vi "Main.vi"(8 "error in (no error)":errorcluster caption="错误输入（无错误）", 11 "人体监测系统 输入":refnum<class "人体健康监测系统.lvclass">) -> (0 "error out":errorcluster caption="错误输出", 3 "人体监测系统 输出":refnum<class "人体健康监测系统.lvclass">)   [LabVIEW 2020, in "人体健康监测系统.lvclass"]
uses:
  OpenUI(Setting).vi
  <vilib>/GPower/VILauncher/Library/Open/OpenByRefnumAndRunFP.vi
  <vilib>/GPower/VILauncher/VILauncher.lvlib
panel:
  in  "OK":bool
  in  "Title":bool
  in  "Title-通讯参数":string="通讯参数"
  out "通讯状态":bool
  in  "Settings":bool
  in  "Title-当前状态":string
  in  "当前状态":string
  in  "Title-模式切换":string="模式切换"
  in  "模式切换":bool
  in  "Title-参数设置":string="参数设置"
  in  "加":bool
  in  "减":bool
  in  "参数设置":bool
  in  "Title-开关机":string="开关机"
  in  "关机":bool
  in  "Title-数据采集和回放":string="数据采集和回放"
  in  "回放文件选择":path
  in  "数据回放":bool
  in  "保存文件名称":string
  in  "停止采集":bool
  in  "开始采集":bool
  out "数据曲线图":waveform(sgl)[](graph)
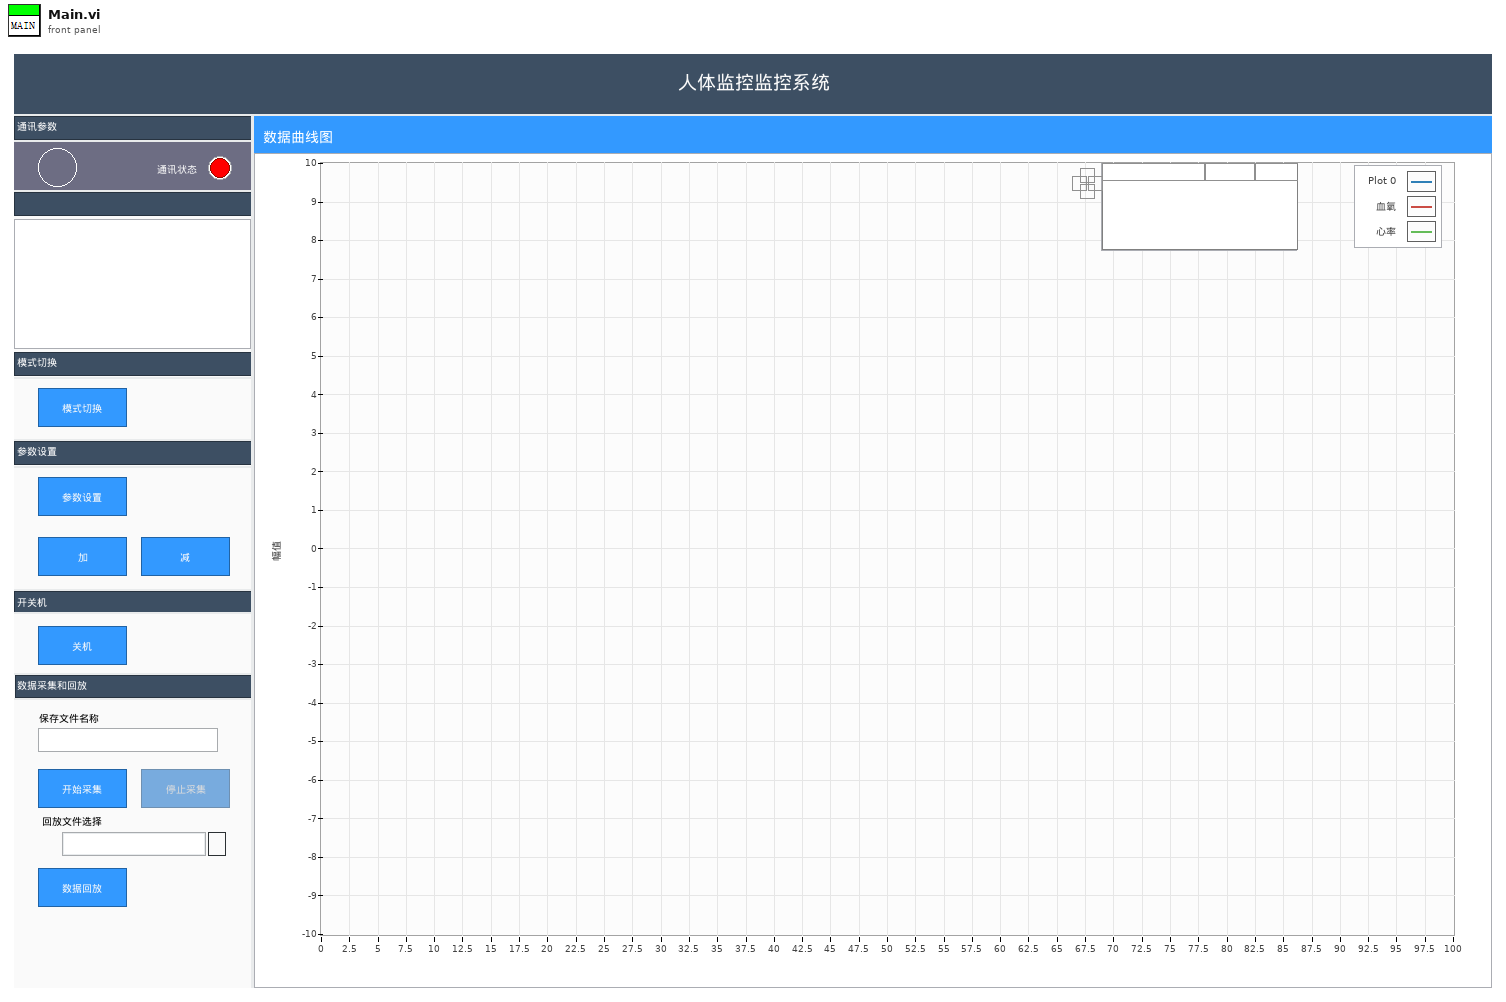
[diagram p1: front panel]
types:
  T1 = enum8{"Enabled", "Disabled", "Disabled and Grayed Out"}
  T2 = enum32{"Invalid", "Standard", "Closed", "Hidden", "Minimized", "Maximized"}
  T3 = enum32{"invalid app kind", "Development System", "Run Time System", "Student Edition", "Embedded LabVIEW", "Evaluation", "Custom"}
  T4 = cluster{"Core":cluster{"Current VI Reference":refnum<vi>, "Close Panel on Exit?":bool}, "Your Boolean data":bool, "Your string data":string, "通讯状态":refnum<vi>, "数据曲线图":refnum<vi>, "Data":waveform(sgl)[], "测试状态？":bool, "开始采集":refnum<vi>, "停止采集":refnum<vi>, "最近三次读取缓存":string[]}
  T5 = cluster{"Current VI Reference":refnum<vi>, "Close Panel on Exit?":bool}
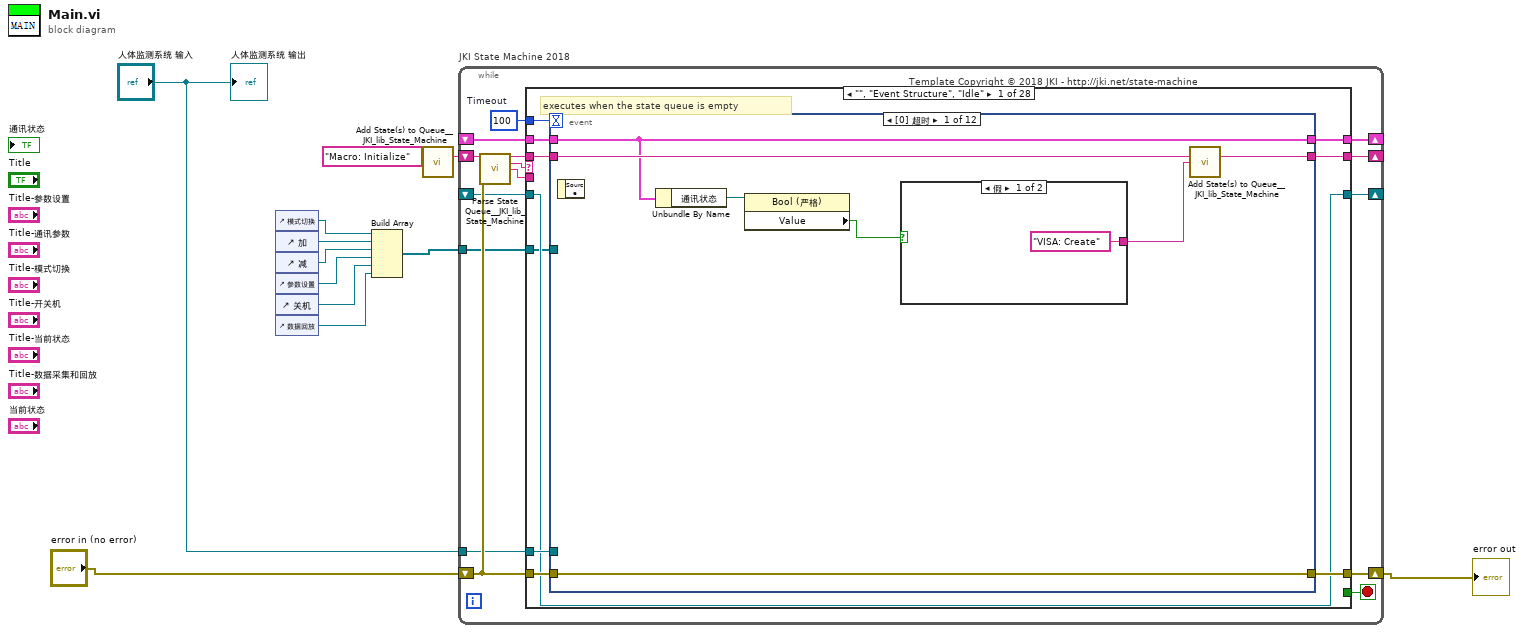
[diagram p0: block diagram]
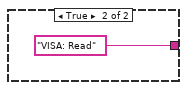
[diagram p2: hidden frame]
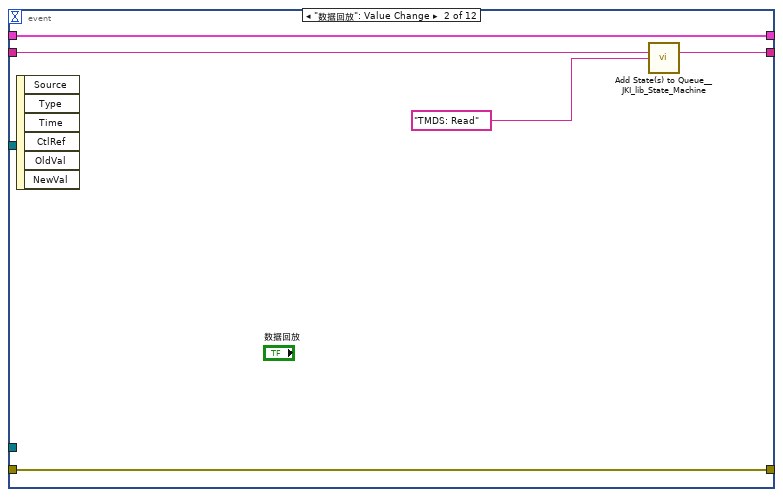
[diagram p3: hidden frame]
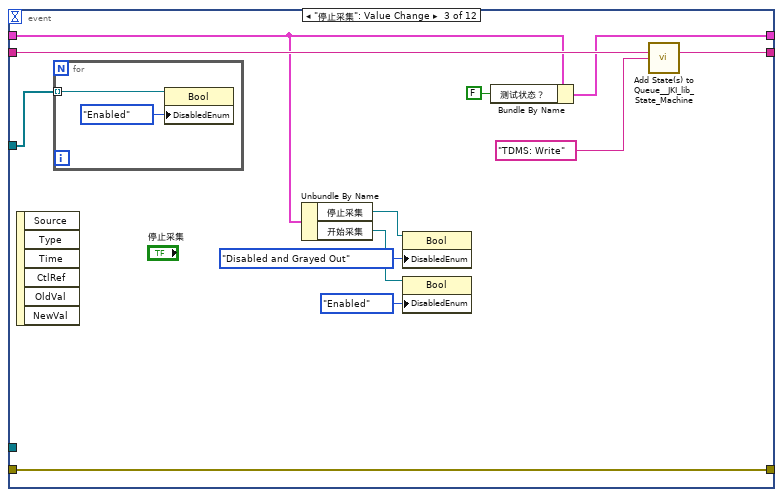
[diagram p4: hidden frame]
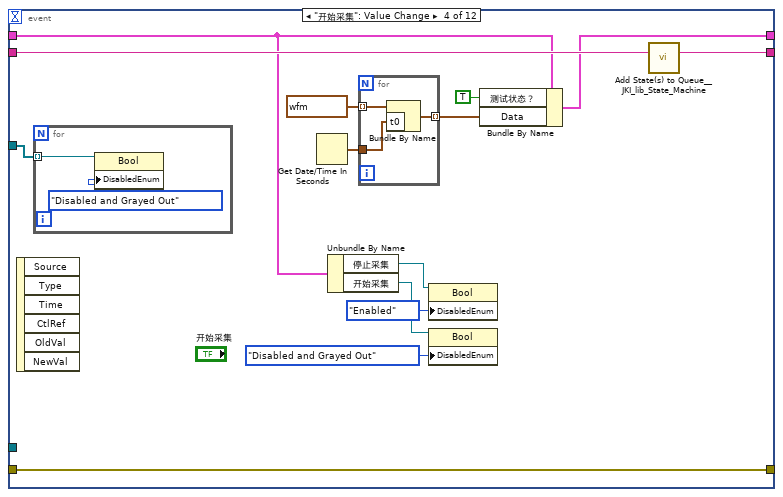
[diagram p5: hidden frame]
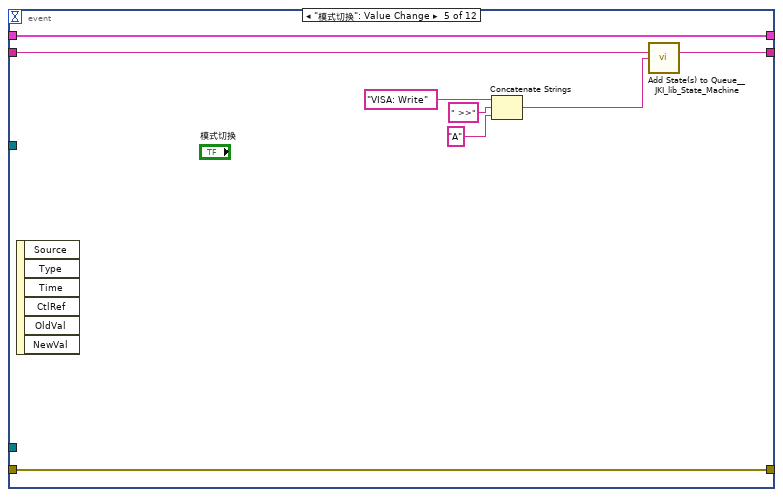
[diagram p6: hidden frame]
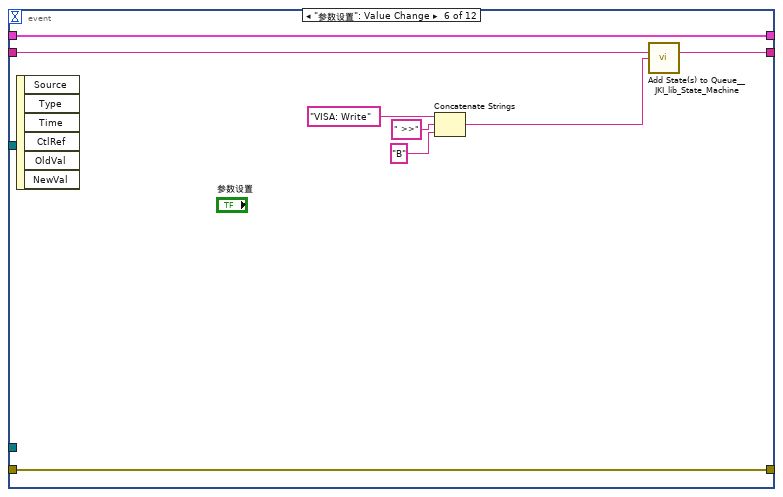
[diagram p7: hidden frame]
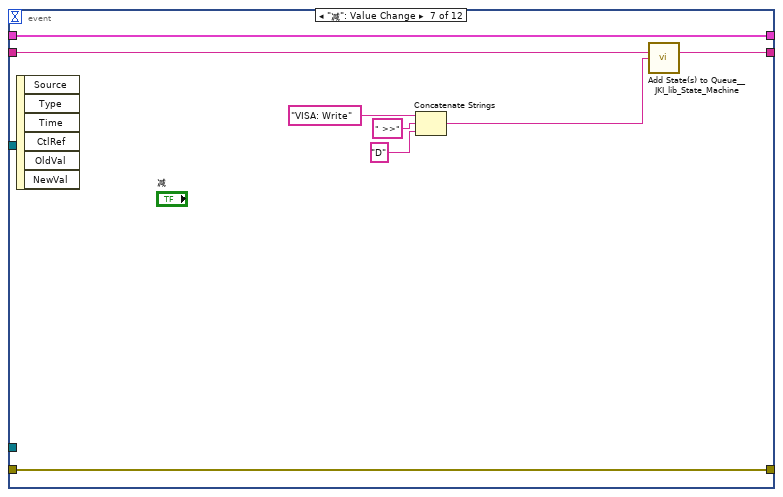
[diagram p8: hidden frame]
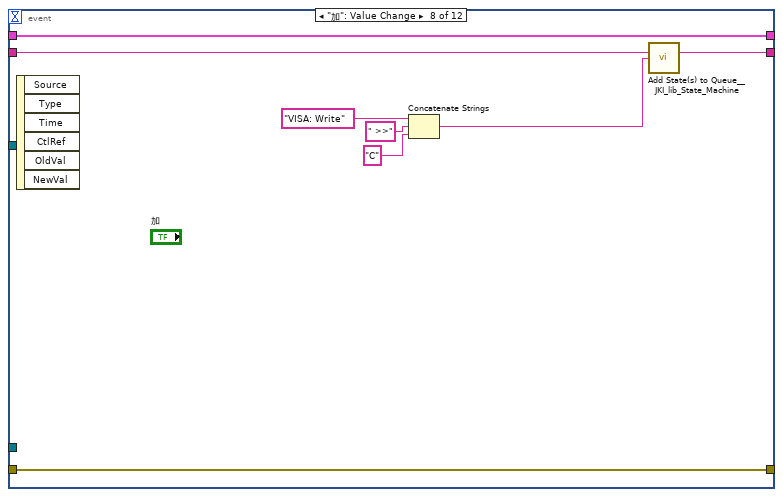
[diagram p9: hidden frame]
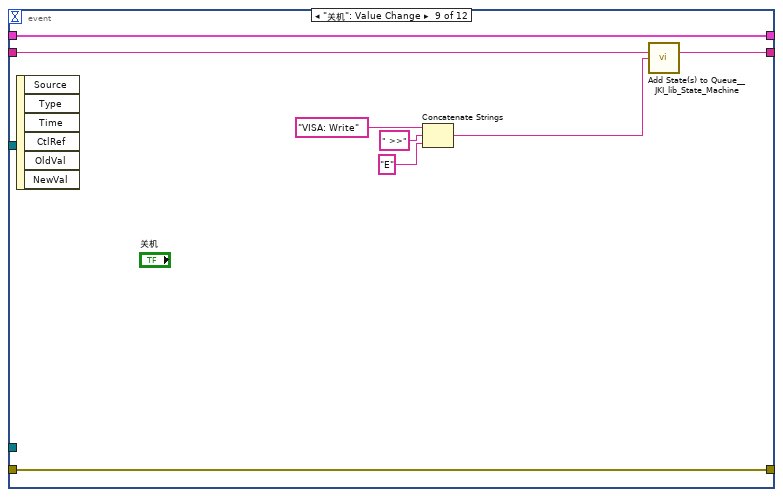
[diagram p10: hidden frame]
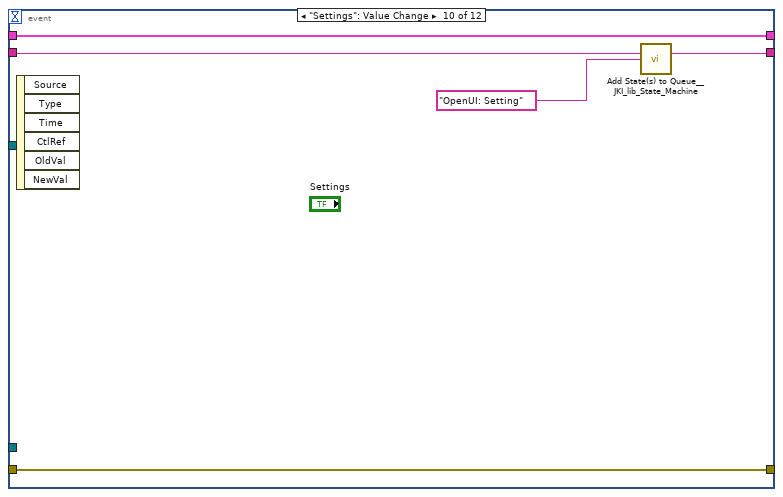
[diagram p11: hidden frame]
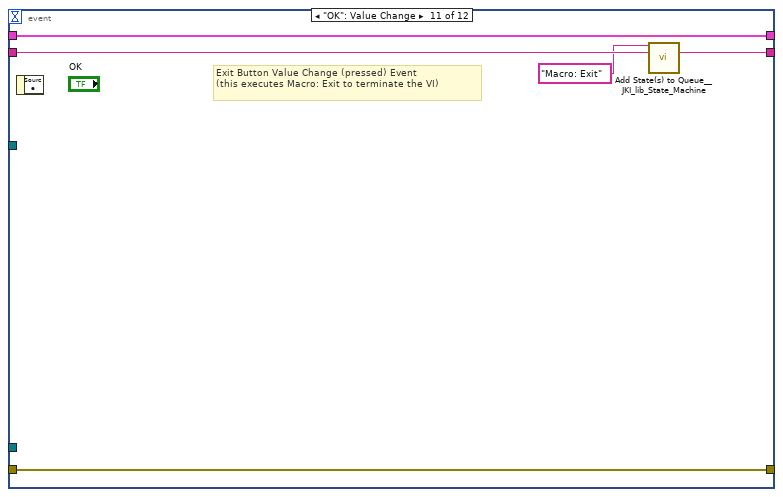
[diagram p12: hidden frame]
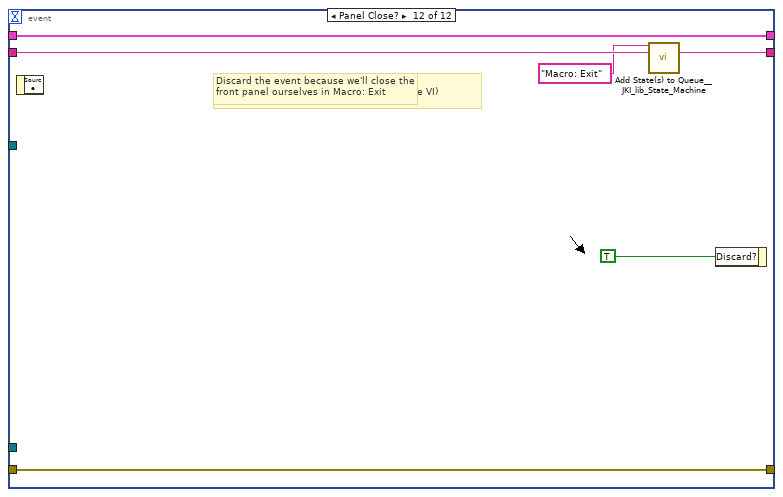
[diagram p13: hidden frame]
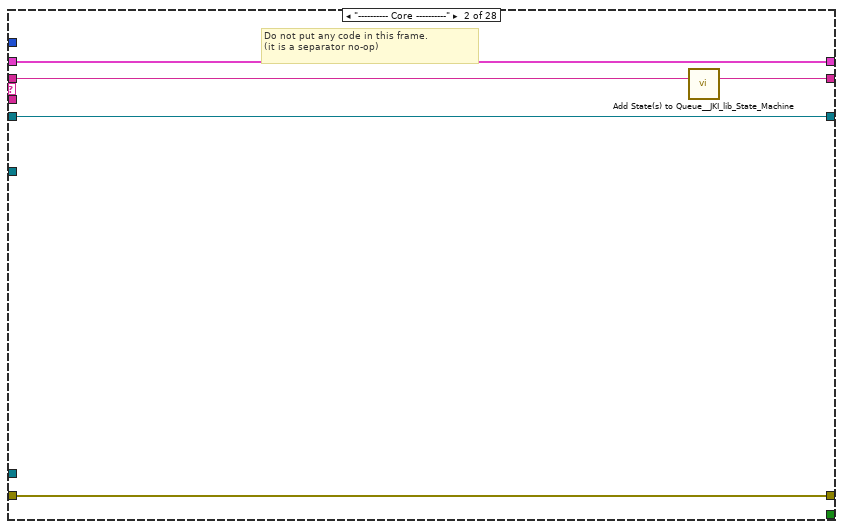
[diagram p14: hidden frame]
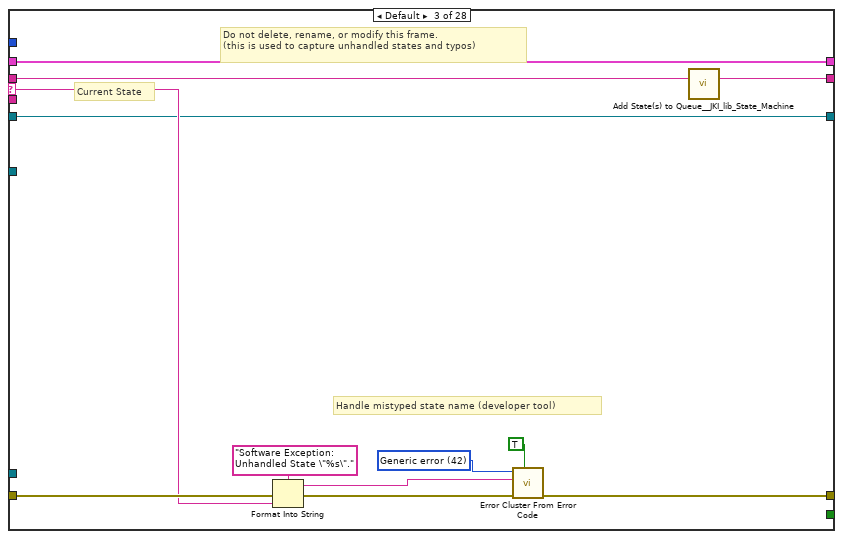
[diagram p15: hidden frame]
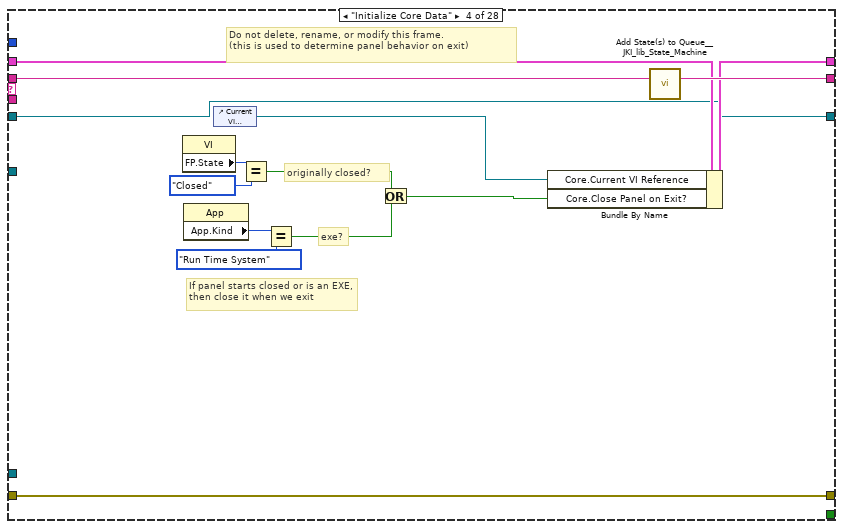
[diagram p16: hidden frame]
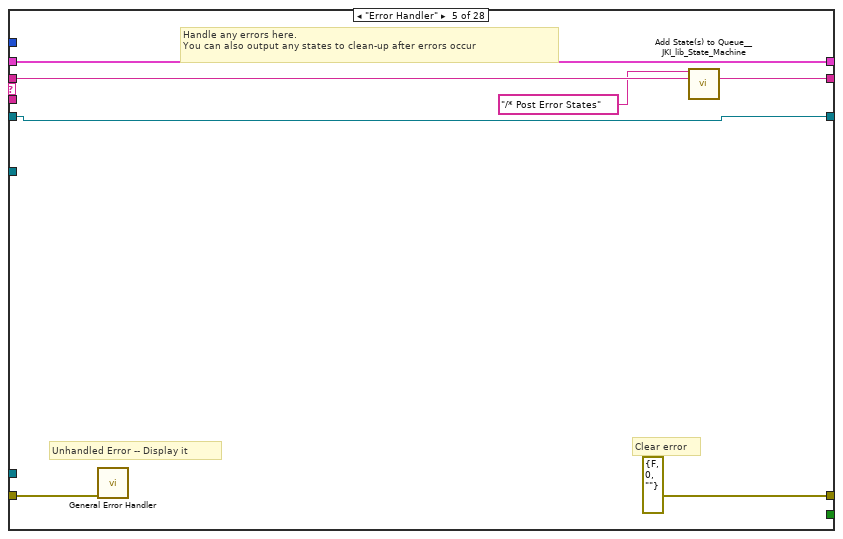
[diagram p17: hidden frame]
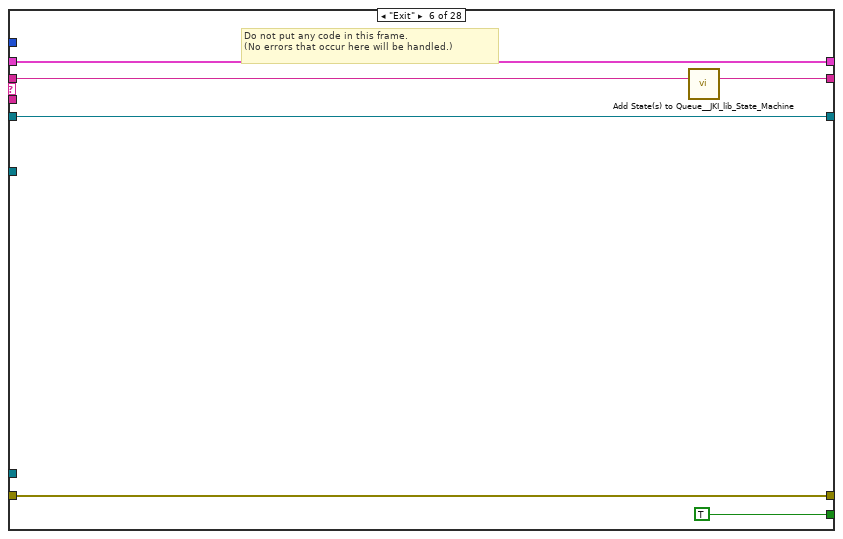
[diagram p18: hidden frame]
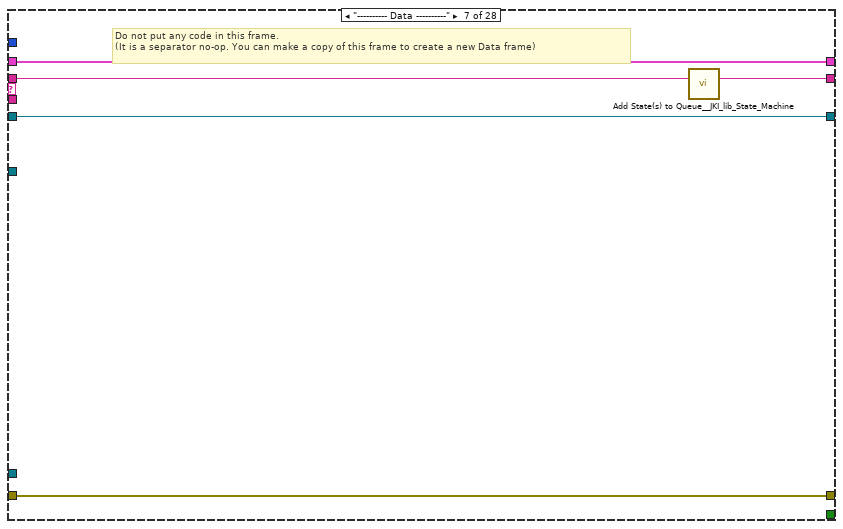
[diagram p19: hidden frame]
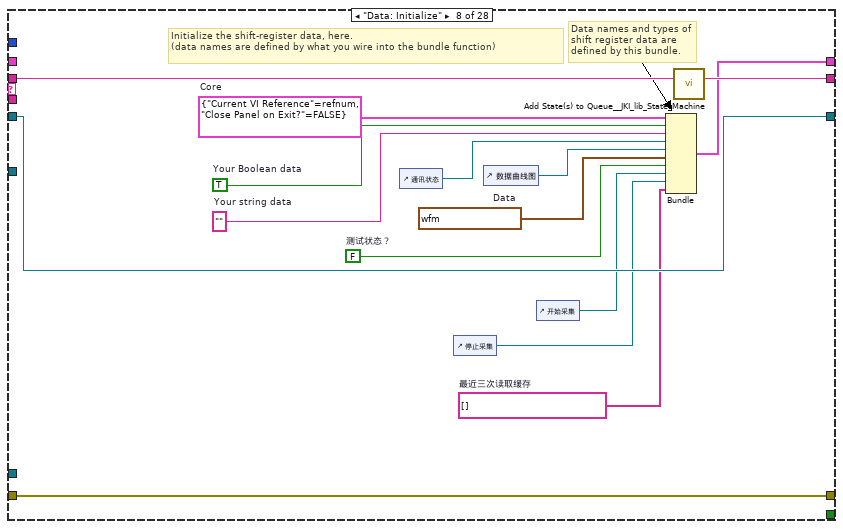
[diagram p20: hidden frame]
diagram:
  n1 = control-ref of="模式切换"() -> (w7:refnum<vi>)
  n2 = control-ref of="加"() -> (w6:refnum<vi>)
  n3 = control-ref of="减"() -> (w5:refnum<vi>)
  n4 = control-ref of="参数设置"() -> (w4:refnum<vi>)
  n5 = control-ref of="关机"() -> (w3:refnum<vi>)
  n6 = control-ref of="数据回放"() -> (w1:refnum<vi>)
  n7 = Build Array(w7, w6, w5, w4, w3, w1) -> (w2:refnum<vi>[])
  n8 = call <vilib>:"Add State(s) to Queue__JKI_lib_State_Machine.vi"("State(s) in (\"\")"="Macro: Initialize") -> ("States Out"=w12:string)  [unwired: 14 in]
  n9 = while "JKI State Machine 2018" {
    shift-right: [w20] -> _
    shift-left: _ -> [w19]
    shift-right: [w23] -> w8
    shift-left: "error in (no error)" -> [w17]
    shift-right: [w22] -> _
    shift-left: w12 -> [w24]
    tunnel: "人体监测系统 输入" -> [w16]
    shift-right: [w15] -> _
    shift-left: _ -> [w14]
    tunnel: w2 -> [w13]
    stop <- w21 stop-if-true
    w18 = 100  # Timeout
    # "Template Copyright © 2018 JKI - http://jki.net/state-machine"
    n10 = call <vilib>:"Parse State Queue__JKI_lib_State_Machine.vi"("State Queue"=w24, "Error In (no error)"=w17) -> ("Remaining States"=w26:string, "Current State"=w27:string, "Arguments"=w25:string)  [unwired: 11 in]
    n11 = case shown="\"\", \"Event Structure\", \"Idle\"" w27 {
      selector: w27 -> [_ _ w147 _ _ _ _ _ _ _ _ _ _ _ _ _ _ _ _ _ _ _ _ _ _ _ _ _]
      tunnel: w26 -> [w37 w145 w151 w171 w178 w184 w189 w204 w211 w216 w227 w236 w248 w318 w324 w337 w342 w349 w354 w359 w367 w376 w401 w413 w421 w429 w434 w443]
      tunnel: w25 -> [_ _ _ _ _ _ _ _ _ _ _ w231 w242 _ _ _ _ _ _ _ w362 _ _ _ _ _ _ _]
      tunnel: w19 -> [w35 w142 w149 w164 w175 w182 w186 _ w206 w213 w219 w234 w244 w315 w321 w335 w339 w347 w351 w356 w365 w371 w386 w410 w419 w427 w431 w437]
      tunnel: [w34 w143 w153 w168 errorcluster {"status"=FALSE, "code"=0, "source"=""} ("error out") w181 w187 w201 w207 w214 w225 w232 w245 w316 w322 w325 w340 w344 w352 w357 w363 w373 w398 w411 w416 w424 w432 w441] -> w23
      tunnel: w17 -> [w33 w143 w152 w168 w174 w181 w187 w201 w208 w214 w225 w233 w246 w316 w322 w327 w340 w345 w352 w357 w364 w374 w399 w411 w417 w425 w432 w441]
      tunnel: [w36 w144 w150 w170 w177 w183 w188 w203 w210 w215 w226 w235 w247 w317 w323 w336 w341 w348 w353 w358 w366 w375 w391 w412 w420 w428 w433 w442] -> w22
      tunnel: [_ _ _ _ _ TRUE _ _ _ _ _ _ _ _ _ _ _ _ _ _ _ _ _ _ _ _ _ _] -> w21
      tunnel: [w32 w142 w149 w169 w175 w182 w186 w202 w206 w213 w219 w234 w244 w315 w321 w335 w339 w347 w351 w356 w365 w371 w385 w410 w419 w427 w431 w436] -> w20
      tunnel: w18 -> [w31 _ _ _ _ _ _ _ _ _ _ _ _ _ _ _ _ _ _ _ _ _ _ _ _ _ _ _]
      tunnel: w16 -> [w30 _ _ _ _ _ _ _ _ _ _ _ _ _ _ _ _ _ _ _ _ _ _ _ _ _ _ _]
      tunnel: [w29 w141 w146 w158 w172 w179 w185 w197 w205 w212 w224 w230 w241 w314 w319 w328 w338 w343 w350 w355 w360 w372 w397 w409 w418 w426 w430 w440] -> w15
      tunnel: w14 -> [w29 w141 w146 w158 w172 w179 w185 w197 w205 w212 w224 w230 w241 w314 w319 w328 w338 w343 w350 w355 w361 _ w400 w409 w418 w426 w430 w440]
      tunnel: w13 -> [w28 _ _ _ _ _ _ _ _ _ w222 _ _ _ _ _ _ _ _ _ _ _ _ _ _ _ _ _]
      frame "", "Event Structure", "Idle" {
        # "executes when the state queue is empty"
        n12 = event shown="[0] 超时" {
          selector: _ -> [_ _ _ _ _ _ _ _ _ _ _ _]
          dyn-events: _ -> [_ _ _ _ _ _ _ _ _ _ _ _]
          timeout: w31 -> [_ _ _ _ _ _ _ _ _ _ _ _]
          tunnel: w37 -> [w44 w51 w63 w79 w92 w100 w108 w116 w124 w126 w134 w140]
          tunnel: [w43 w50 w62 w78 w91 w99 w107 w115 w123 w127 w133 w139] -> w36
          tunnel: w35 -> [w41 w48 w54 w66 w89 w97 w105 w113 w121 w129 w131 w137]
          tunnel: [w42 w49 w61 w77 w90 w98 w106 w114 w122 w128 w132 w138] -> w34
          tunnel: w33 -> [w42 w49 w61 w77 w90 w98 w106 w114 w122 w128 w132 w138]
          tunnel: [w41 w48 w59 w72 w89 w97 w105 w113 w121 w129 w131 w137] -> w32
          tunnel: w30 -> [_ _ _ _ _ _ _ _ _ _ _ _]
          tunnel: w28 -> [_ _ w57 w71 _ _ _ _ _ _ _ _]
          event Timeout {
            n13 = event-data() -> ()  [unwired: 1 in, 1 out]
            n14 = Unbundle By Name(w41) -> ("通讯状态"=w40:refnum<vi>)
            n15 = property class="Bool (严格)"(reference=w40) -> ("Value"=w39:bool)  [unwired: 1 in, 2 out]
            n16 = case shown="假" w39 {
              tunnel: ["VISA: Create" ("State(s) at Back (\"\")") "VISA: Read" ("State(s) at Back (\"\")")] -> w38
              frame False {
              }
              frame True {
              }
            }
            n17 = call <vilib>:"Add State(s) to Queue__JKI_lib_State_Machine.vi"("State(s) in (\"\")"=w44, "State(s) at Back (\"\")"=w38) -> ("States Out"=w43:string)  [unwired: 13 in]
          }
          event "数据回放": Value Change {
            n18 = event-data() -> ()  [unwired: 1 in, 6 out]
            n19 = call <vilib>:"Add State(s) to Queue__JKI_lib_State_Machine.vi"("State(s) in (\"\")"=w51, "State(s) at Back (\"\")"="TMDS: Read" ("State(s) at Back (\"\")")) -> ("States Out"=w50:string)  [unwired: 13 in]
          }
          event "停止采集": Value Change {
            n20 = event-data() -> ()  [unwired: 1 in, 6 out]
            n21 = for {
              tunnel: w57 -> [w65] mode=indexing
              n22 = property class="Bool"(reference=w65, "DisabledEnum"=T1."Enabled" ("禁用")) -> ()  [unwired: 1 in, 2 out]
            }
            n23 = Unbundle By Name(w54) -> ("停止采集"=w56:refnum<vi>, "开始采集"=w53:refnum<vi>)
            n24 = property class="Bool"(reference=w56, "DisabledEnum"=T1."Disabled and Grayed Out" ("禁用")) -> ()  [unwired: 1 in, 2 out]
            n25 = property class="Bool"(reference=w53, "DisabledEnum"=T1."Enabled" ("禁用")) -> ()  [unwired: 1 in, 2 out]
            n26 = Bundle By Name(cluster=w54, "测试状态？"=FALSE) -> (w59:T4)
            n27 = call <vilib>:"Add State(s) to Queue__JKI_lib_State_Machine.vi"("State(s) in (\"\")"=w63, "State(s) at Back (\"\")"="TDMS: Write" ("State(s) at Back (\"\")")) -> ("States Out"=w62:string)  [unwired: 13 in]
          }
          event "开始采集": Value Change {
            n28 = event-data() -> ()  [unwired: 1 in, 6 out]
            n29 = for {
              tunnel: w71 -> [w81] mode=indexing
              n30 = property class="Bool"(reference=w81, "DisabledEnum"=T1."Disabled and Grayed Out" ("禁用")) -> ()  [unwired: 1 in, 2 out]
            }
            n31 = Get Date/Time In Seconds() -> (seconds since 1Jan1904=w74:timestamp)
            n32 = Unbundle By Name(w66) -> ("停止采集"=w70:refnum<vi>, "开始采集"=w68:refnum<vi>)
            n33 = for {
              tunnel: waveform(sgl)[] [{"t0"=timestamp(0 s since 1904-01-01), "dt"=1.0, "Y"=[]}, {"t0"=timestamp(0 s since 1904-01-01), "dt"=1.0, "Y"=[]}, {"t0"=timestamp(0 s since 1904-01-01), "dt"=1.0, "Y"=[]}] ("Data") -> [w84] mode=indexing
              tunnel: w74 -> [w83]
              tunnel: [w82] -> w73 mode=indexing
              n34 = Bundle By Name(cluster=w84, "t0"=w83) -> (w82:waveform(sgl))
            }
            n35 = property class="Bool"(reference=w70, "DisabledEnum"=T1."Enabled" ("禁用")) -> ()  [unwired: 1 in, 2 out]
            n36 = property class="Bool"(reference=w68, "DisabledEnum"=T1."Disabled and Grayed Out" ("禁用")) -> ()  [unwired: 1 in, 2 out]
            n37 = Bundle By Name(cluster=w66, "测试状态？"=TRUE, "Data"=w73) -> (w72:T4)
            n38 = call <vilib>:"Add State(s) to Queue__JKI_lib_State_Machine.vi"("State(s) in (\"\")"=w79) -> ("States Out"=w78:string)  [unwired: 14 in]
          }
          event "模式切换": Value Change {
            n39 = event-data() -> ()  [unwired: 1 in, 6 out]
            n40 = Concatenate Strings("VISA: Write" ("字符串"), " >>" ("字符串"), "A" ("字符串")) -> (w85:string)
            n41 = call <vilib>:"Add State(s) to Queue__JKI_lib_State_Machine.vi"("State(s) in (\"\")"=w92, "State(s) at Back (\"\")"=w85) -> ("States Out"=w91:string)  [unwired: 13 in]
          }
          event "参数设置": Value Change {
            n42 = event-data() -> ()  [unwired: 1 in, 6 out]
            n43 = Concatenate Strings("VISA: Write" ("字符串"), " >>" ("字符串"), "B" ("字符串")) -> (w93:string)
            n44 = call <vilib>:"Add State(s) to Queue__JKI_lib_State_Machine.vi"("State(s) in (\"\")"=w100, "State(s) at Back (\"\")"=w93) -> ("States Out"=w99:string)  [unwired: 13 in]
          }
          event "减": Value Change {
            n45 = event-data() -> ()  [unwired: 1 in, 6 out]
            n46 = Concatenate Strings("VISA: Write" ("字符串"), " >>" ("字符串"), "D" ("字符串")) -> (w101:string)
            n47 = call <vilib>:"Add State(s) to Queue__JKI_lib_State_Machine.vi"("State(s) in (\"\")"=w108, "State(s) at Back (\"\")"=w101) -> ("States Out"=w107:string)  [unwired: 13 in]
          }
          event "加": Value Change {
            n48 = event-data() -> ()  [unwired: 1 in, 6 out]
            n49 = Concatenate Strings("VISA: Write" ("字符串"), " >>" ("字符串"), "C" ("字符串")) -> (w109:string)
            n50 = call <vilib>:"Add State(s) to Queue__JKI_lib_State_Machine.vi"("State(s) in (\"\")"=w116, "State(s) at Back (\"\")"=w109) -> ("States Out"=w115:string)  [unwired: 13 in]
          }
          event "关机": Value Change {
            n51 = event-data() -> ()  [unwired: 1 in, 6 out]
            n52 = Concatenate Strings("VISA: Write" ("字符串"), " >>" ("字符串"), "E" ("字符串")) -> (w117:string)
            n53 = call <vilib>:"Add State(s) to Queue__JKI_lib_State_Machine.vi"("State(s) in (\"\")"=w124, "State(s) at Back (\"\")"=w117) -> ("States Out"=w123:string)  [unwired: 13 in]
          }
          event "Settings": Value Change {
            n54 = event-data() -> ()  [unwired: 1 in, 6 out]
            n55 = call <vilib>:"Add State(s) to Queue__JKI_lib_State_Machine.vi"("State(s) in (\"\")"=w126, "State(s) at Back (\"\")"="OpenUI: Setting" ("State(s) at Back (\"\")")) -> ("States Out"=w127:string)  [unwired: 13 in]
          }
          event "OK": Value Change {
            # "Exit Button Value Change (pressed) Event\n(this executes Macro: Exit to terminate the VI)"
            n56 = event-data() -> ()  [unwired: 1 in, 1 out]
            n57 = call <vilib>:"Add State(s) to Queue__JKI_lib_State_Machine.vi"("State(s) in Front (\"\")"="Macro: Exit", "State(s) in (\"\")"=w134) -> ("States Out"=w133:string)  [unwired: 13 in]
          }
          event Panel Close? {
            # "Discard the event because we'll close the front panel ourselves in Macro: Exit"
            # "Close Panel button (pressed) Event\n(this executes Macro: Exit to terminate the VI)"
            n58 = event-data() -> ()  [unwired: 1 in, 1 out]
            n59 = call <vilib>:"Add State(s) to Queue__JKI_lib_State_Machine.vi"("State(s) in Front (\"\")"="Macro: Exit", "State(s) in (\"\")"=w140) -> ("States Out"=w139:string)  [unwired: 13 in]
            n60 = event-data("Discard?"=TRUE) -> ()  [unwired: 1 in, 1 out]
          }
        }
      }
      frame "---------- Core ----------" {
        # "Do not put any code in this frame.\n(it is a separator no-op)"
        n61 = call <vilib>:"Add State(s) to Queue__JKI_lib_State_Machine.vi"("State(s) in (\"\")"=w145) -> ("States Out"=w144:string)  [unwired: 14 in]
      }
      frame Default {
        w156 = 42 items=["No error", "Argument error", "Memory is full", "Out of zone", "End of file", "File already open", "Generic file I/O error", "File not found", "File permission error", "Disk is full", "Duplicate path", "Too many files open", "System feature not enabled", "Resource file not found", "Cannot add resource", "Resource not found", "Image not found", "Image memory error", "Pen does not exist", "Config type invalid", "Config token not found", "Config parse error", "Config memory error", "Bad external code format", "Bad external code offset", "External code not present", "Null window", "Destroy window error", "Null menu", "Print aborted", "Bad print record", "Print driver error", "Windows error during printing", "Memory error during printing", "Print dialog error", "Generic print error", "Invalid device refnum", "Device not found", "Device parameter error", "Device unit error", "Cannot open device", "Device call aborted", "Generic error", "Cancelled by user", "Object ID too low", "Object ID too high", "Object not in heap", "Unknown heap", "Unknown object (invalid DefProc)", "Unknown object (DefProc not in table)", "Message out of range", "Invalid (null) method", "Unknown message", "Manager call not supported", "Bad address", "Network operation in progress", "Network operation timed out", "Connection is busy", "Network attribute not supported", "Network error", "Address in use", "System out of memory", "Connection aborted", "Connection refused", "Not connected", "Already connected", "Connection closed", "Initialization error (interapplication manager)", "Bad occurrence", "Wait on unbound occurrence handler", "Occurrence queue overflow", "Datalog type conflict", "Unused", "Unrecognized type (interapplication manager)", "Memory corrupt", "Failed to make temporary DLL", "Old CIN version", "Drag socket not found", "Failed to load drop-object", "Failed to register OLE object", "Failed to release OLE object", "Format specifier type mismatch", "Unknown format specifier", "Too few format specifiers", "Too many format specifiers", "Scan failed", "Newer CIN version", "Error converting to variant", "Runtime menu error", "Password tampered", "Variant attribute not found", "Incompatible variant data type", "Event data is not available", "Event Store is not present", "Occurrence is not found", "Event Queue is not created", "Event info is not available", "Refnum passed is NULL", "Error retrieving Class GUID", "Error retrieving CoClass GUID", "Error retrieving TypeLib GUID.", "Bad built application magic bytes.", "Specific driver is different from the specific driver associated with the Logical Name.", "There is no session opened to the class driver.", "Max Error", "MAX - Error with config objects", "MAX - Error loading configuration", "MAX - Group not supported"]
        # "Current State"
        # "Do not delete, rename, or modify this frame.\n(this is used to capture unhandled states and typos)"
        # "Handle mistyped state name (developer tool)"
        n62 = Format Into String(format string="Software Exception: Unhandled State \"%s\"." ("message"), error in=w152, w147) -> (resulting string=w155:string, error out=w154:errorcluster)  [unwired: 1 in]
        n63 = call <vilib>:"Error Cluster From Error Code.vi"("show call chain? (False)"=TRUE, "error in (no error)"=w154, "error message (\"\")"=w155, "error code (0)"=w156) -> ("error out"=w153:errorcluster)  [unwired: 5 in]
        n64 = call <vilib>:"Add State(s) to Queue__JKI_lib_State_Machine.vi"("State(s) in (\"\")"=w151) -> ("States Out"=w150:string)  [unwired: 14 in]
      }
      frame "Initialize Core Data" {
        # "Do not delete, rename, or modify this frame.\n(this is used to determine panel behavior on exit)"
        # "originally closed?"
        # "exe?"
        # "If panel starts closed or is an EXE, then close it when we exit"
        n65 = property class="VI"() -> ("FP.State"=w161:T2)  [unwired: 2 in, 2 out]
        n66 = property class="App"() -> ("App.Kind"=w167:T3)  [unwired: 2 in, 2 out]
        n67 = control-ref of="Current VI Reference"() -> (w162:refnum<vi>)
        n68 = Equal?(x=w161, y=T2."Closed" ("Front Panel Window:State")) -> (x = y?=w159:bool)
        n69 = Equal?(x=w167, y=T3."Run Time System" ("Application:Kind")) -> (x = y?=w165:bool)
        n70 = Or(x=w159, y=w165) -> (x .or. y?=w163:bool)
        n71 = Bundle By Name(cluster=w164, "Core.Current VI Reference"=w162, "Core.Close Panel on Exit?"=w163) -> (w169:T4)
        n72 = call <vilib>:"Add State(s) to Queue__JKI_lib_State_Machine.vi"("State(s) in (\"\")"=w171) -> ("States Out"=w170:string)  [unwired: 14 in]
      }
      frame "Error Handler" {
        # "Unhandled Error -- Display it"
        # "Handle any errors here.\nYou can also output any states to clean-up after errors occur"
        # "Clear error"
        n73 = call <vilib>:"General Error Handler.vi"("error in (no error)"=w174) -> ()  [unwired: 10 in, 5 out]
        n74 = call <vilib>:"Add State(s) to Queue__JKI_lib_State_Machine.vi"("State(s) in Front (\"\")"="/* Post Error States", "State(s) in (\"\")"=w178) -> ("States Out"=w177:string)  [unwired: 13 in]
      }
      frame "Exit" {
        # "Do not put any code in this frame.\n(No errors that occur here will be handled.)"
        n75 = call <vilib>:"Add State(s) to Queue__JKI_lib_State_Machine.vi"("State(s) in (\"\")"=w184) -> ("States Out"=w183:string)  [unwired: 14 in]
      }
      frame "---------- Data ----------" {
        # "Do not put any code in this frame.\n(It is a separator no-op. You can make a copy of this frame to create a new Data frame)"
        n76 = call <vilib>:"Add State(s) to Queue__JKI_lib_State_Machine.vi"("State(s) in (\"\")"=w189) -> ("States Out"=w188:string)  [unwired: 14 in]
      }
      frame "Data: Initialize" {
        w190 = string[] []  # 最近三次读取缓存
        w193 = FALSE  # 测试状态？
        w194 = waveform(sgl)[] [{"t0"=timestamp(0 s since 1904-01-01), "dt"=1.0, "Y"=[]}, {"t0"=timestamp(0 s since 1904-01-01), "dt"=1.0, "Y"=[]}, {"t0"=timestamp(0 s since 1904-01-01), "dt"=1.0, "Y"=[]}]  # Data
        w198 = T5 {"Current VI Reference"=refnum, "Close Panel on Exit?"=FALSE}  # Core
        w200 = TRUE  # Your Boolean data
        w199 = ""  # Your string data
        # "Data names and types of shift register data are defined by this bundle."
        # "Initialize the shift-register data, here.\n(data names are defined by what you wire into the bundle function)"
        n77 = control-ref of="通讯状态"() -> (w196:refnum<vi>)
        n78 = control-ref of="停止采集"() -> (w191:refnum<vi>)
        n79 = control-ref of="数据曲线图"() -> (w195:refnum<vi>)
        n80 = control-ref of="开始采集"() -> (w192:refnum<vi>)
        n81 = Bundle("Core"=w198, "Your Boolean data"=w200, "Your string data"=w199, "通讯状态"=w196, "数据曲线图"=w195, "Data"=w194, "测试状态？"=w193, "开始采集"=w192, "停止采集"=w191, "最近三次读取缓存"=w190) -> (w202:T4)  [unwired: 1 in]
        n82 = call <vilib>:"Add State(s) to Queue__JKI_lib_State_Machine.vi"("State(s) in (\"\")"=w204) -> ("States Out"=w203:string)  [unwired: 14 in]
      }
      frame "Data: Cleanup" {
        # "Cleanup any data and references, here.\n(this is called automatically, by the Macro: Exit)"
        n83 = Unbundle By Name(w206) -> ("Core.Current VI Reference"=w209:refnum<vi>)
        n84 = Close Reference(reference=w209, error in (no error)=w208) -> (error out=w207:errorcluster)
        n85 = call <vilib>:"Add State(s) to Queue__JKI_lib_State_Machine.vi"("State(s) in (\"\")"=w211) -> ("States Out"=w210:string)  [unwired: 14 in]
      }
      frame "---------- UI ----------" {
        # "Do not put any code in this frame.\n(It is a separator no-op. You can make a copy of this frame to create a new UI frame)"
        n86 = call <vilib>:"Add State(s) to Queue__JKI_lib_State_Machine.vi"("State(s) in (\"\")"=w216) -> ("States Out"=w215:string)  [unwired: 14 in]
      }
      frame "UI: Initialize" {
        n87 = for {
          tunnel: w222 -> [w229] mode=indexing
          n88 = property class="Bool"(reference=w229, "DisabledEnum"=T1."Enabled" ("禁用")) -> ()  [unwired: 1 in, 2 out]
        }
        n89 = Unbundle By Name(w219) -> ("开始采集"=w218:refnum<vi>, "停止采集"=w221:refnum<vi>)
        n90 = property class="Bool"(reference=w221, "DisabledEnum"=T1."Disabled and Grayed Out" ("禁用")) -> ()  [unwired: 1 in, 2 out]
        n91 = property class="Bool"(reference=w218, "DisabledEnum"=T1."Enabled" ("禁用")) -> ()  [unwired: 1 in, 2 out]
        n92 = call <vilib>:"Add State(s) to Queue__JKI_lib_State_Machine.vi"("State(s) in (\"\")"=w227, "State(s) at Back (\"\")"="VISA: Create" ("State(s) at Back (\"\")")) -> ("States Out"=w226:string)  [unwired: 13 in]
      }
      frame "UI: Cursor Set" {
        # "Argument"
        # "Set and Unset Cursor Busy.\n(Usage: \"UI: Cursor Set >> Busy|Idle\")"
        n93 = case shown="\"Idle\", 默认" w231 {
          tunnel: w233 -> [w238 w240]
          tunnel: [w237 w239] -> w232
          frame "Idle", Default {
            n94 = call <vilib>:"Unset Busy.vi"("error in (no error)"=w238) -> ("error out"=w237:errorcluster)  [unwired: 10 in]
          }
          frame "Busy" {
            n95 = call <vilib>:"Set Busy.vi"("error in (no error)"=w240) -> ("error out"=w239:errorcluster)  [unwired: 9 in, 1 out]
          }
        }
        n96 = call <vilib>:"Add State(s) to Queue__JKI_lib_State_Machine.vi"("State(s) in (\"\")"=w236) -> ("States Out"=w235:string)  [unwired: 14 in]
      }
      frame "UI: Front Panel State" {
        # "Argument"
        # "Set Front Panel Open or Closed\n(Usage: \"UI: Front Panel State >> Open|Close\")"
        n97 = Unbundle By Name(w244) -> ("Core.Current VI Reference"=w243:refnum<vi>)
        n98 = case shown="\"Minimize\", \"Minimized\"" w242 {
          tunnel: w246 -> [w254 w269 w280 w293 w306]
          tunnel: [w256 w270 w282 w295 w308] -> w245
          tunnel: w243 -> [w255 w267 w281 w294 w307]
          frame "Open", "Standard", Default {
            w249 = T2."Standard" ("State")
            n99 = property class="VI"(reference=w255, error in=w254) -> (reference out=w252:refnum<vi>, error out=w253:errorcluster, "FP.State"=w251:T2)
            n100 = Not Equal?(x=w251, y=w249) -> (x != y?=w250:bool)
            n101 = case shown="真" w250 {
              tunnel: [w260 w262] -> w256
              tunnel: w253 -> [w259 w262]
              tunnel: w252 -> [w258 _]
              tunnel: w249 -> [w257 _]
              frame True {
                n102 = invoke class="VI" method="FP.Open"(reference=w258, error in=w259, "Activate"=TRUE, "State"=w257) -> (error out=w260:errorcluster)  [unwired: 1 in, 4 out]
              }
              frame False {
              }
            }
          }
          frame "Close", "Closed" {
            n103 = property class="VI"(reference=w267, error in=w269) -> (reference out=w266:refnum<vi>, error out=w268:errorcluster, "FP.State"=w264:T2)
            n104 = Not Equal?(x=w264, y=T2."Closed" ("Front Panel Window:State")) -> (x != y?=w263:bool)
            n105 = case shown="真" w263 {
              tunnel: [w271 w274] -> w270
              tunnel: w268 -> [w271 w273]
              tunnel: w266 -> [_ w272]
              frame False {
              }
              frame True {
                n106 = invoke class="VI" method="FP.Close"(reference=w272, error in=w273) -> (error out=w274:errorcluster)  [unwired: 1 in, 2 out]
              }
            }
          }
          frame "Hidden", "Hide" {
            w275 = T2."Hidden" ("State")
            n107 = property class="VI"(reference=w281, error in=w280) -> (reference out=w278:refnum<vi>, error out=w279:errorcluster, "FP.State"=w277:T2)
            n108 = Not Equal?(x=w277, y=w275) -> (x != y?=w276:bool)
            n109 = case shown="真" w276 {
              tunnel: [w286 w287] -> w282
              tunnel: w279 -> [w285 w287]
              tunnel: w278 -> [w284 _]
              tunnel: w275 -> [w283 _]
              frame True {
                n110 = invoke class="VI" method="FP.Open"(reference=w284, error in=w285, "State"=w283) -> (error out=w286:errorcluster)  [unwired: 2 in, 4 out]
              }
              frame False {
              }
            }
          }
          frame "Minimize", "Minimized" {
            w288 = T2."Minimized" ("State")
            n111 = property class="VI"(reference=w294, error in=w293) -> (reference out=w291:refnum<vi>, error out=w292:errorcluster, "FP.State"=w290:T2)
            n112 = Not Equal?(x=w290, y=w288) -> (x != y?=w289:bool)
            n113 = case shown="真" w289 {
              tunnel: [w299 w300] -> w295
              tunnel: w292 -> [w298 w300]
              tunnel: w291 -> [w297 _]
              tunnel: w288 -> [w296 _]
              frame True {
                n114 = invoke class="VI" method="FP.Open"(reference=w297, error in=w298, "State"=w296) -> (error out=w299:errorcluster)  [unwired: 2 in, 4 out]
              }
              frame False {
              }
            }
          }
          frame "Maximize", "Maximized" {
            w301 = T2."Maximized" ("State")
            n115 = property class="VI"(reference=w307, error in=w306) -> (reference out=w304:refnum<vi>, error out=w305:errorcluster, "FP.State"=w303:T2)
            n116 = Not Equal?(x=w303, y=w301) -> (x != y?=w302:bool)
            n117 = case shown="真" w302 {
              tunnel: [w312 w313] -> w308
              tunnel: w305 -> [w311 w313]
              tunnel: w304 -> [w310 _]
              tunnel: w301 -> [w309 _]
              frame True {
                n118 = invoke class="VI" method="FP.Open"(reference=w310, error in=w311, "State"=w309) -> (error out=w312:errorcluster)  [unwired: 2 in, 4 out]
              }
              frame False {
              }
            }
          }
        }
        n119 = call <vilib>:"Add State(s) to Queue__JKI_lib_State_Machine.vi"("State(s) in (\"\")"=w248) -> ("States Out"=w247:string)  [unwired: 14 in]
      }
      frame "---------- Macro ----------" {
        # "Do not put any code in this frame.\n(It is a separator no-op. You can make a copy of this frame to create a new Macro frame)"
        n120 = call <vilib>:"Add State(s) to Queue__JKI_lib_State_Machine.vi"("State(s) in (\"\")"=w318) -> ("States Out"=w317:string)  [unwired: 14 in]
      }
      frame "Macro: Initialize" {
        w320 = "Data: Initialize\nInitialize Core Data\nUI: Initialize\nUI: Front Panel State >> Open"  # Data: Initialize Initialize Core Data UI: Initialize UI: Front Panel State >> Open
        # "Initialization Macro\n(This is called once, when the VI starts)"
        n121 = call <vilib>:"Add State(s) to Queue__JKI_lib_State_Machine.vi"("State(s) in Front (\"\")"=w320, "State(s) in (\"\")"=w324) -> ("States Out"=w323:string)  [unwired: 13 in]
      }
      frame "Macro: Exit" {
        # "Exit Macro\n(This is called once, when the VI exits)"
        n122 = Unbundle By Name(w335) -> ("Core.Close Panel on Exit?"=w334:bool)
        n123 = VISA Close(VISA resource name=w328, error in (no error)=w327) -> (error out=w326:errorcluster)
        n124 = call <vilib>:"Clear Errors.vi"("error in (no error)"=w326) -> ("error out"=w325:errorcluster)  [unwired: 5 in, 1 out]
        n125 = Select(t="UI: Front Panel State >> Close", s=w334, f="") -> (s? t:f=w331:string)
        n126 = call <vilib>:"Add State(s) to Queue__JKI_lib_State_Machine.vi"("State(s) in (\"\")"=w331, "State(s) at Back (\"\")"="Data: Cleanup\nExit") -> ("States Out"=w329:string)  [unwired: 13 in]
        n127 = call <vilib>:"Add State(s) to Queue__JKI_lib_State_Machine.vi"("State(s) in Front (\"\")"=w329, "State(s) in (\"\")"=w337) -> ("States Out"=w336:string)  [unwired: 13 in]
      }
      frame "---------- OpenUI ----------" {
        # "Template Separator\n(You can make a copy of, or modify, this frame)"
        n128 = call <vilib>:"Add State(s) to Queue__JKI_lib_State_Machine.vi"("State(s) in (\"\")"=w342) -> ("States Out"=w341:string)  [unwired: 14 in]
      }
      frame "OpenUI: Setting" {
        # "Your code here.\n(You can make a copy of, or modify, this frame)"
        n129 = vi-ref "人体健康监测系统.lvclass:OpenUI(Setting).vi"() -> (w346:refnum<vi>)
        n130 = call-poly <vilib>:"OpenAndRun.vi"("VI refnum"=w346, "Error in"=w345) -> ("Error out"=w344:errorcluster)  [unwired: 7 in, 6 out]
        n131 = call <vilib>:"Add State(s) to Queue__JKI_lib_State_Machine.vi"("State(s) in (\"\")"=w349) -> ("States Out"=w348:string)  [unwired: 14 in]
      }
      frame "New Category: 2" {
        # "Your code here.\n(You can make a copy of, or modify, this frame)"
        n132 = call <vilib>:"Add State(s) to Queue__JKI_lib_State_Machine.vi"("State(s) in (\"\")"=w354) -> ("States Out"=w353:string)  [unwired: 14 in]
      }
      frame "---------- VISA ----------" {
        # "Template Separator\n(You can make a copy of, or modify, this frame)"
        n133 = call <vilib>:"Add State(s) to Queue__JKI_lib_State_Machine.vi"("State(s) in (\"\")"=w359) -> ("States Out"=w358:string)  [unwired: 14 in]
      }
      frame "VISA: Write" {
        # "Template Separator\n(You can make a copy of, or modify, this frame)"
        n134 = call "VISA(Write).vi"("error in (no error)"=w364, "写入缓冲区"=w362, "VISA资源名称"=w361) -> ("error out"=w363:errorcluster, "VISA资源名称输出"=w360:refnum<visa-resource-name>)  [unwired: 7 in]
        n135 = call <vilib>:"Add State(s) to Queue__JKI_lib_State_Machine.vi"("State(s) in (\"\")"=w367) -> ("States Out"=w366:string)  [unwired: 14 in]
      }
      frame "VISA: Create" {
        # "Template Separator\n(You can make a copy of, or modify, this frame)"
        n136 = Unbundle By Name(w371) -> ("通讯状态"=w370:refnum<vi>)
        n137 = call "VISA(Create).vi"("error in (no error)"=w374) -> ("error out"=w373:errorcluster, "F?"=w369:bool, "VISA resource name out"=w372:refnum<visa-resource-name>)  [unwired: 8 in]
        n138 = Not(x=w369) -> (.not. x?=w368:bool)
        n139 = property class="Bool (严格)"(reference=w370, "Value"=w368) -> ()  [unwired: 1 in, 2 out]
        n140 = call <vilib>:"Add State(s) to Queue__JKI_lib_State_Machine.vi"("State(s) in (\"\")"=w376) -> ("States Out"=w375:string)  [unwired: 14 in]
      }
      frame "VISA: Read" {
        # "Template Separator\n(You can make a copy of, or modify, this frame)"
        n141 = Unbundle By Name(w386) -> ("测试状态？"=w390:bool, "通讯状态"=w394:refnum<vi>, "最近三次读取缓存"=w377:string[])
        n142 = call "VISA(Read).vi"("error in (no error)"=w399, "VISA资源名称"=w400) -> ("error out"=w398:errorcluster, "F？"=w395:bool, "读取缓冲区"=w384:string, "VISA资源名称"=w397:refnum<visa-resource-name>, "x != 0?"=w392:bool)  [unwired: 5 in]
        n143 = Not(x=w395) -> (.not. x?=w396:bool)
        n144 = property class="Bool (严格)"(reference=w394, "Value"=w396) -> ()  [unwired: 1 in, 2 out]
        n145 = local read "当前状态"() -> (w393:string)
        n146 = case shown="真" w392 {
          tunnel: w384 -> [_ w408]
          tunnel: w393 -> [_ w407]
          tunnel: [FALSE ("更新曲线") w405] -> w389
          tunnel: w377 -> [_ w404]
          frame False {
          }
          frame True {
            n147 = call "Data(Analysis).vi"("当前状态"=w407, "读取缓冲区"=w408, "最近三次读取缓存"=w404) -> ("当前状态"=w406:string, "更新曲线"=w405:bool)  [unwired: 6 in]
            n148 = local write "当前状态"(w406) -> ()
          }
        }
        n149 = And(x=w390, y=w389) -> (x .and. y?=w388:bool)
        n150 = case shown="真" w388 {
          tunnel: [_ "Graph: Read" ("State(s) at Back (\"\")")] -> w387
          frame False {
          }
          frame True {
          }
        }
        n151 = Insert Into Array(array=w377, new element=w384) -> (w383:string[])  [unwired: 1 in]
        n152 = Array Size(array=w383) -> (size(s)=w382:i32)
        n153 = Subtract(x=w382, y=3) -> (x-y=w380:i32)
        n154 = Array Subset(array=w383, index=w380, length=3 ("长度")) -> (w378:string[])
        n155 = call <vilib>:"Add State(s) to Queue__JKI_lib_State_Machine.vi"("State(s) in (\"\")"=w401, "State(s) at Back (\"\")"=w387) -> ("States Out"=w391:string)  [unwired: 13 in]
        n156 = Bundle By Name(cluster=w386, "最近三次读取缓存"=w378) -> (w385:T4)
      }
      frame "---------- TDMS ----------" {
        # "Template Separator\n(You can make a copy of, or modify, this frame)"
        n157 = call <vilib>:"Add State(s) to Queue__JKI_lib_State_Machine.vi"("State(s) in (\"\")"=w413) -> ("States Out"=w412:string)  [unwired: 14 in]
      }
      frame "TMDS: Read" {
        # "Template Separator\n(You can make a copy of, or modify, this frame)"
        n158 = call "TDMS(Read).vi"("error in (no error)"=w417, "文件路径"="回放文件选择") -> ("error out"=w416:errorcluster, "数据"=→"数据曲线图":waveform(sgl)[])  [unwired: 7 in, 1 out]
        n159 = call <vilib>:"Add State(s) to Queue__JKI_lib_State_Machine.vi"("State(s) in (\"\")"=w421) -> ("States Out"=w420:string)  [unwired: 14 in]
      }
      frame "TDMS: Write" {
        # "Template Separator\n(You can make a copy of, or modify, this frame)"
        n160 = local read "数据曲线图"() -> (w422:waveform(sgl)[])
        n161 = call "TDMS(Write).vi"("error in (no error)"=w425, "数据"=w422, "保存文件名称"="保存文件名称") -> ("error out"=w424:errorcluster)  [unwired: 8 in]
        n162 = call <vilib>:"Add State(s) to Queue__JKI_lib_State_Machine.vi"("State(s) in (\"\")"=w429) -> ("States Out"=w428:string)  [unwired: 14 in]
      }
      frame "---------- Graph ----------" {
        # "Template Separator\n(You can make a copy of, or modify, this frame)"
        n163 = call <vilib>:"Add State(s) to Queue__JKI_lib_State_Machine.vi"("State(s) in (\"\")"=w434) -> ("States Out"=w433:string)  [unwired: 14 in]
      }
      frame "Graph: Read" {
        n164 = local read "当前状态"() -> (w438:string)
        n165 = Unbundle By Name(w437) -> ("Data"=w439:waveform(sgl)[])
        n166 = call "Data(String to Data).vi"("当前状态"=w438, "数据"=w439) -> ("数组"=w435:waveform(sgl)[])  [unwired: 9 in]
        n167 = Bundle By Name(cluster=w437, "Data"=w435) -> (w436:T4)
        n168 = local write "数据曲线图"(w435) -> ()
        n169 = call <vilib>:"Add State(s) to Queue__JKI_lib_State_Machine.vi"("State(s) in (\"\")"=w443) -> ("States Out"=w442:string)  [unwired: 14 in]
      }
    }
  }
  "error out" <- w8
  "人体监测系统 输出" <- "人体监测系统 输入"
